vi "GetWl.vi"(0 "VISA resource name":refnum<visa-resource-name>="COM3", 5 "error in (no error)":errorcluster) -> (14 "VISA resource name out":refnum<visa-resource-name>, 16 "Wavelength":dbl format="%#_7g", 19 "error out":errorcluster)   [LabVIEW 2016]
doc: "Function: tga1240_config_pulse\n\nPurpose: Configure the parameters for a pulse waveform"
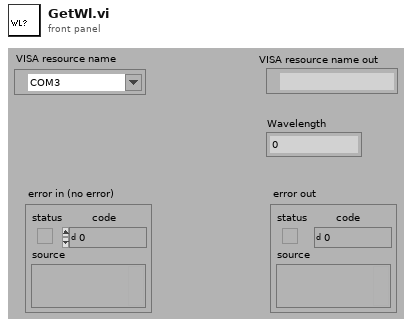
[diagram p1: front panel]
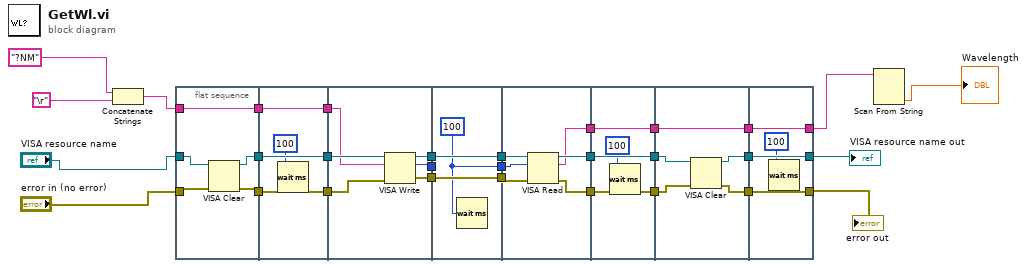
[diagram p0: block diagram]
diagram:
  n1 = Concatenate Strings("?NM" ("format string"), "\r") -> (w20:string)
  n2 = flat-sequence {
    tunnel: w20 -> [w35]
    tunnel: "error in (no error)" -> [w31]
    tunnel: "VISA resource name" -> [w34]
    tunnel: [w33] -> w15
    tunnel: [w32] -> w13
    tunnel: [w35] -> w11
    tunnel: w15 -> [w39]
    tunnel: [w39] -> w14
    tunnel: w13 -> [w38]
    tunnel: [w38] -> w12
    tunnel: w11 -> [w37]
    tunnel: [w37] -> w10
    tunnel: [w42] -> w28
    tunnel: [w41] -> w27
    tunnel: [w40] -> w26
    tunnel: w14 -> [w45]
    tunnel: w12 -> [w44]
    tunnel: w10 -> [w43]
    tunnel: w28 -> [w48]
    tunnel: w27 -> [w47]
    tunnel: [w48] -> w25
    tunnel: [w47] -> w24
    tunnel: w26 -> [_]
    tunnel: [w46] -> w23
    tunnel: w25 -> [w51]
    tunnel: w24 -> [w52]
    tunnel: w23 -> [w49]
    tunnel: [w54] -> w9
    tunnel: [w53] -> w7
    tunnel: [w50] -> w5
    tunnel: w9 -> [w58]
    tunnel: [w58] -> w8
    tunnel: w7 -> [w57]
    tunnel: [w57] -> w6
    tunnel: w5 -> [w56]
    tunnel: [w56] -> w4
    tunnel: w8 -> [w63]
    tunnel: w6 -> [w62]
    tunnel: w4 -> [w59]
    tunnel: [w61] -> w3
    tunnel: [w60] -> w2
    tunnel: [w59] -> w1
    tunnel: [w65] -> w16
    tunnel: [w66] -> w18
    tunnel: [w67] -> w19
    tunnel: w3 -> [w67]
    tunnel: w2 -> [w66]
    tunnel: w1 -> [w65]
    frame #0 {
      n3 = VISA Clear(VISA resource name=w34, error in (no error)=w31) -> (VISA resource name out=w33:refnum<visa-resource-name>, error out=w32:errorcluster)
    }
    frame #1 {
      n4 = Wait (ms)(milliseconds to wait=100) -> ()  [unwired: 1 out]
    }
    frame #2 {
      n5 = VISA Write(VISA resource name=w45, write buffer=w43, error in (no error)=w44) -> (VISA resource name out=w42:refnum<visa-resource-name>, return count=w40:u32, error out=w41:errorcluster)
    }
    frame #3 {
      w46 = 100
      n6 = Wait (ms)(milliseconds to wait=w46) -> ()  [unwired: 1 out]
    }
    frame #4 {
      n7 = VISA Read(VISA resource name=w51, byte count=w49, error in (no error)=w52) -> (VISA resource name out=w54:refnum<visa-resource-name>, read buffer=w50:string, error out=w53:errorcluster)  [unwired: 1 out]
    }
    frame #5 {
      n8 = Wait (ms)(milliseconds to wait=100) -> ()  [unwired: 1 out]
    }
    frame #6 {
      n9 = VISA Clear(VISA resource name=w63, error in (no error)=w62) -> (VISA resource name out=w61:refnum<visa-resource-name>, error out=w60:errorcluster)
    }
    frame #7 {
      n10 = Wait (ms)(milliseconds to wait=100) -> ()  [unwired: 1 out]
    }
  }
  n11 = Scan From String(input string=w16) -> (output 1=→"Wavelength":dbl)  [unwired: 4 in, 3 out]
  "error out" <- w18
  "VISA resource name out" <- w19
